vi "ifNanUseLastValue.vi"(1 "Starting value":dbl, 2 "Number":dbl) -> (0 "Latest num. value":dbl)   [LabVIEW 2014]
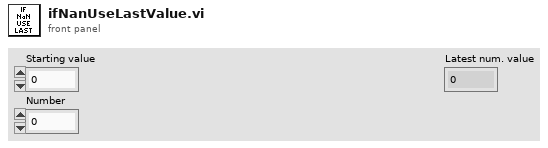
[diagram p1: front panel]
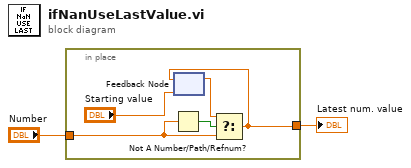
[diagram p0: block diagram]
diagram:
  n1 = in-place {
    in-place-border: "Number" -> [w4]
    in-place-border: [w6] -> w1
    n2 = Not A Number/Path/Refnum?(number/path/refnum=w4) -> (NaN/Path/Refnum?=w7:bool)
    n3 = feedback #1("Starting value") -> (w5:dbl)
    n4 = Select(t=w5, s=w7, f=w4) -> (s? t:f=w6:dbl)
    n5 = feedback-in #1(w6) -> ()
  }
  "Latest num. value" <- w1
